vi "Save Config.vi"(7 "Clear Changes (T)":bool=TRUE, 8 "error in (no error)":errorcluster, 10 "Storage":refnum<class "Config Storage.lvclass">, 11 "Config Manager in":refnum<class "Config Manager.lvclass">) -> (0 "error out":errorcluster, 3 "Config Manager out":refnum<class "Config Manager.lvclass">)   [LabVIEW 2020, in "CDM-Config.lvlib" / "Config Manager.lvclass"]
uses:
  Config Manager.lvclass
  Config Storage/Config Storage.lvclass
  Config Manager.lvclass/Config Manager.ctl
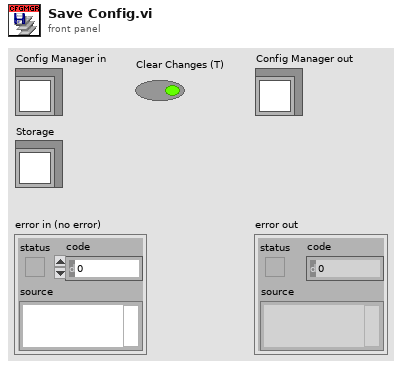
[diagram p1: front panel]
types:
  T1 = typedef "CDM-Config.lvlib/Config Manager.lvclass/Ref Data.ctl" = cluster{"Elements":refnum<class "Config Element.lvclass">[], "Name Separator":string, "Hierarchy Map":map{string[], i32}, "Meta Name Map":map{string, i32[]}, "Element Map":map{refnum<class "Config Element.lvclass">, i32}, "Changed":bool[]}
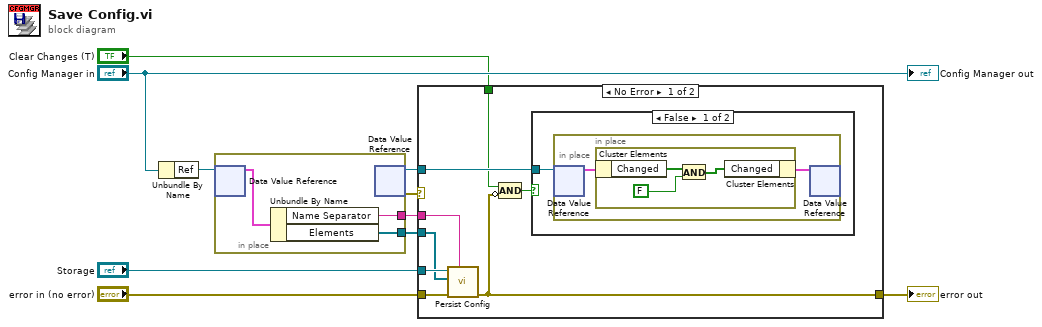
[diagram p0: block diagram]
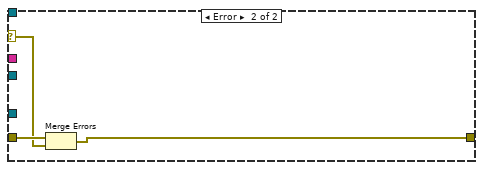
[diagram p3: hidden frame]
diagram:
  n1 = Unbundle By Name("Config Manager in") -> ("Ref"=w10:refnum<data-value>)
  n2 = in-place {
    in-place-border: [w12] -> w7
    in-place-border: [w11] -> w5
    n3 = in-place-dvr #1(w10) -> (w13:T1)  [unwired: 1 out]
    n4 = Unbundle By Name(w13) -> ("Name Separator"=w11:string, "Elements"=w12:refnum<class "Config Element.lvclass">[])
    n5 = in-place-dvr #1() -> (w3:refnum<data-value>, w1:errorcluster)  [unwired: 1 in]
  }
  n6 = case shown="No Error" w1 {
    selector: w1 -> [_ w29]
    tunnel: "Storage" -> [w21 _]
    tunnel: w7 -> [w20 _]
    tunnel: "error in (no error)" -> [w19 w30]
    tunnel: w5 -> [w18 _]
    tunnel: [w17 w28] -> w4
    tunnel: w3 -> [w16 _]
    tunnel: "Clear Changes (T)" -> [w14 _]
    frame No Error {
      n7 = call-dynamic "Persist Config.vi"("Name Delimiter"=w18, "error in (no error)"=w19, "Elements"=w20, "Config Storage in"=w21) -> ("error out"=w17:errorcluster)  [unwired: 6 in, 1 out]
      n8 = Compound Arithmetic op=AND(w14, invert w17) -> (w15:bool)
      n9 = case shown="False" w15 {
        tunnel: w16 -> [w22 _]
        frame False {
          n10 = in-place {
            n11 = in-place-dvr #2(w22) -> (w24:T1)  [unwired: 1 out]
            n12 = in-place {
              n13 = in-place-cluster #3(w24) -> ("Changed"=w27:bool[])
              n14 = And(x=w27, y=FALSE) -> (x .and. y?=w25:bool[])
              n15 = in-place-cluster #3("Changed"=w25) -> (w23:T1)
            }
            n16 = in-place-dvr #2(w23) -> ()  [unwired: 2 out]
          }
        }
        frame True {
        }
      }
    }
    frame Error {
      n17 = Merge Errors(w30, w29) -> (w28:errorcluster)
    }
  }
  "error out" <- w4
  "Config Manager out" <- "Config Manager in"
